vi "导出校准测试数据.vi"(7 "阀值":dbl, 8 "error in":errorcluster, 9 "COM":i32=4, 11 "IN":i32=129) -> (0 "error out":errorcluster)   [LabVIEW 2015]
uses:
  <vilib>/addons/_office/excel.llb/Excel Easy Table (str).vi
  server/Global/SeverGlobal.vi
  <vilib>/Utility/NIReport.llb/NI_report.lvclass
  <vilib>/Utility/NIReport.llb/Excel/NI_Excel.lvclass
  <vilib>/addons/_office/NI_ReportGenerationToolkit.lvlib
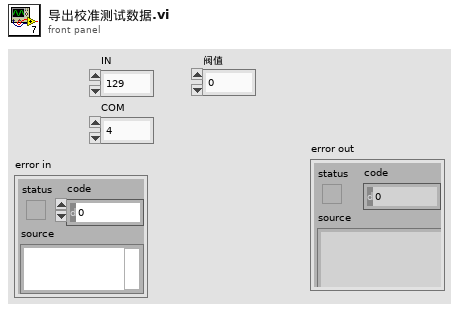
[diagram p1: front panel]
types:
  T1 = enum16{"Standard Report", "HTML", "Word", "Excel"}
  T2 = enum16{"maximized", "minimized", "normal", "no change"}
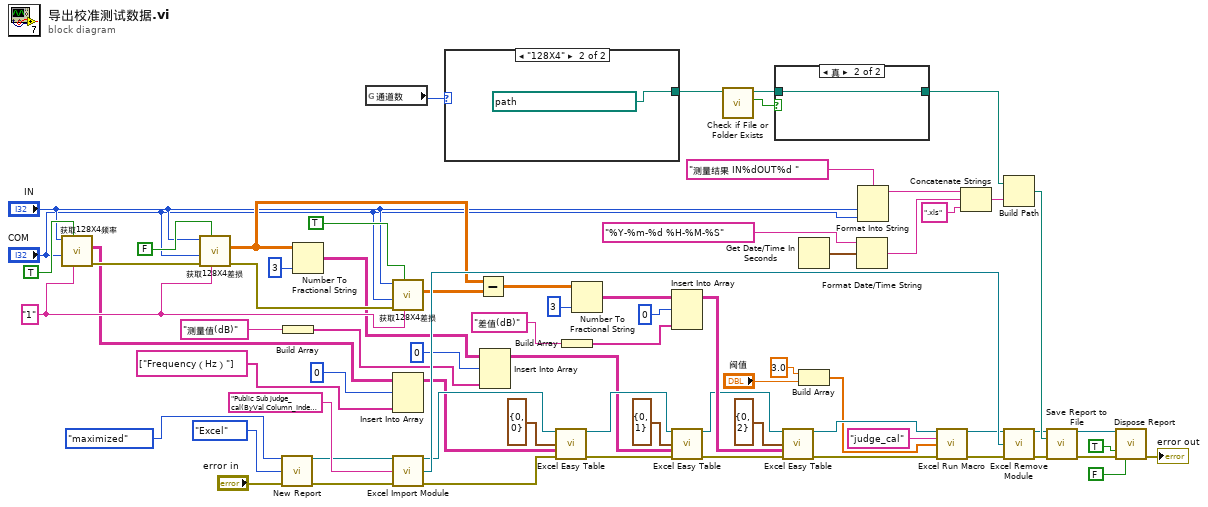
[diagram p0: block diagram]
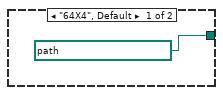
[diagram p2: hidden frame]
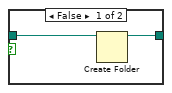
[diagram p3: hidden frame]
diagram:
  w38 = "1" ("testType")
  n1 = call "获取128X4频率.vi"("testType"=w38, "ref"=TRUE, "COM"="COM", "A"="IN") -> ("error out"=w40:errorcluster, "Freq&S21"=w35:string[][])  [unwired: 6 in]
  n2 = call "获取128X4差损.vi"("testType"=w38, "ref"=FALSE, "error in (no error)"=w40, "COM"="COM", "A"="IN") -> ("error out"=w50:errorcluster, "S21"=w25:dbl[][])  [unwired: 5 in]
  n3 = call <vilib>:"New Report.vi"("window state (normal)"=T2."maximized", "report type"=T1."Excel", "error in (no error)"="error in") -> ("report out"=w10:refnum<class "NI_report.lvclass">, "error out"=w9:errorcluster)  [unwired: 11 in]
  n4 = Build Array("测量值(dB)" ("format string")) -> (w21:string[])
  n5 = Number To Fractional String(number=w25, precision (6)=i16 3) -> (F-format string=w23:string[][])  [unwired: 2 in]
  n6 = global read "SeverGlobal.vi" "通道数"() -> (w2:enum16{"64X4", "128X4"})
  n7 = call "获取128X4差损.vi"("testType"=w38, "ref"=TRUE, "error in (no error)"=w50, "COM"="COM", "A"="IN") -> ("S21"=w47:dbl[][])  [unwired: 5 in, 1 out]
  n8 = Insert Into Array(array=w35, index (row)=0, new element=string[] ["Frequency（Hz）"] ("new element/subarray")) -> (w32:string[][])  [unwired: 1 in]
  n9 = call <vilib>:"Excel Import Module.vi"("report in"=w10, "module code (\"\")"="Public Sub judge_cal(ByVal Column_Index As Single, ByVal limit As Single)\n    Dim iRows, i As Integer\n    Dim formu As String\n    Dim loc As Range\n    Dim letter As String\n    iRows = ActiveSheet.UsedRange.Rows.Count\n    For i = 2 To iRows\n        letter = VBA.Split(Cells(1, Column_Index).Address, \"$\")(1)\n        Set loc = Range(letter & i)\n        If abs(loc.Value) > limit Then\n            loc.Font.Color = -16776961\n        End If\n    Next\nEnd Sub" ("module code (\"\")"), "error in (no error)"=w9) -> ("report out"=w36:refnum<class "NI_report.lvclass">, "module reference"=w67:refnum<k7>, "error out"=w11:errorcluster)  [unwired: 10 in]
  n10 = case shown="\"128X4\"" w2 {
    tunnel: [path "D:/64X4数据/基准数据" ("base path") path "D:/128X4数据/基准数据" ("base path")] -> w1
    frame "64X4", Default {
    }
    frame "128X4" {
    }
  }
  n11 = Subtract(x=w25, y=w47) -> (x-y=w46:dbl[][])
  n12 = Insert Into Array(array=w23, index (row)=0, new element=w21) -> (w20:string[][])  [unwired: 1 in]
  n13 = call-poly <vilib>:"Excel Easy Table.vi"("report in"=w36, "start (0, 0)"=cluster{"row":i32, "column":i32} {"row"=0, "column"=0}, "text data"=w32, "error in (no error)"=w11) -> ("report out"=w30:refnum<class "NI_report.lvclass">, "error out"=w29:errorcluster)  [unwired: 7 in, 3 out]
  n14 = Build Array("差值(dB)" ("format string")) -> (w42:string[])
  n15 = Number To Fractional String(number=w46, precision (6)=i16 3) -> (F-format string=w44:string[][])  [unwired: 2 in]
  n16 = Insert Into Array(array=w44, index (row)=0, new element=w42) -> (w31:string[][])  [unwired: 1 in]
  n17 = call-poly <vilib>:"Excel Easy Table.vi"("report in"=w30, "start (0, 0)"=cluster{"row":i32, "column":i32} {"row"=0, "column"=1}, "text data"=w20, "error in (no error)"=w29) -> ("report out"=w19:refnum<class "NI_report.lvclass">, "error out"=w18:errorcluster)  [unwired: 7 in, 3 out]
  n18 = call <vilib>:"Check if File or Folder Exists.vi"("path"=w1) -> ("file or folder exists?"=w59:bool, "dup path"=w60:path)  [unwired: 8 in, 1 out]
  n19 = case shown="真" w59 {
    tunnel: w60 -> [w75 w76]
    tunnel: [w74 w76] -> w61
    frame False {
      n20 = Create Folder(path (use dialog)=w75) -> (created path=w74:path)  [unwired: 2 in, 2 out]
    }
    frame True {
    }
  }
  n21 = call-poly <vilib>:"Excel Easy Table.vi"("report in"=w19, "start (0, 0)"=cluster{"row":i32, "column":i32} {"row"=0, "column"=2}, "text data"=w31, "error in (no error)"=w18) -> ("report out"=w16:refnum<class "NI_report.lvclass">, "error out"=w17:errorcluster)  [unwired: 7 in, 3 out]
  n22 = Get Date/Time In Seconds() -> (seconds since 1Jan1904=w58:timestamp)
  n23 = Build Array(3.0 ("element"), "阀值") -> (w14:dbl[])
  n24 = Format Date/Time String(time format string (%c)="%Y-%m-%d %H-%M-%S", seconds (now)=w58) -> (date/time string=w55:string)  [unwired: 1 in]
  n25 = Format Into String(format string="测量结果 IN%dOUT%d ", "IN", "COM") -> (resulting string=w3:string)  [unwired: 2 in, 1 out]
  n26 = call <vilib>:"Excel Run Macro.vi"("report in"=w16, "macro name"="judge_cal", "parameters"=w14, "error in (no error)"=w17) -> ("report out"=w8:refnum<class "NI_report.lvclass">, "error out"=w7:errorcluster)  [unwired: 9 in, 1 out]
  n27 = Concatenate Strings(w3, w55, ".xls") -> (w54:string)
  n28 = Build Path(base path=w61, name or relative path=w54) -> (appended path=w53:path)
  n29 = call <vilib>:"Excel Remove Module.vi"("report in"=w8, "module reference"=w67, "error in (no error)"=w7) -> ("report out"=w52:refnum<class "NI_report.lvclass">, "error out"=w51:errorcluster)  [unwired: 11 in]
  n30 = call-dynamic "Save Report to File.vi"("report in"=w52, "report file path"=w53, "error in (no error)"=w51) -> ("report out"=w66:refnum<class "NI_report.lvclass">, "error out"=w65:errorcluster)  [unwired: 11 in]
  n31 = call-dynamic "Dispose Report.vi"("report in"=w66, "save changes? (F)"=TRUE, "error in (no error)"=w65, "close report? (T)"=FALSE) -> ("error out"=→"error out":errorcluster)  [unwired: 11 in]
